vi "final with visa and without stepper motor.vi"() -> ()   [LabVIEW 2022 SP3]
uses:
  <vilib>/DAQmx/create/channels.llb/DAQmx Create Channel (AI-Voltage-Basic).vi
  <vilib>/DAQmx/read.llb/DAQmx Read (Analog 1D DBL NChan 1Samp).vi
panel:
  in  "VISA resource name 2":refnum<visa-resource-name>
  in  "VISA resource name":refnum<visa-resource-name>
  in  "physical channels":tag
  in  "stop":bool
  out "humidity":dbl
  in  "Voltage":dbl
  out "?":bool
  out "Counter":dbl
  out "number":dbl
  out "weight":dbl
  out "voltage (weight)":dbl
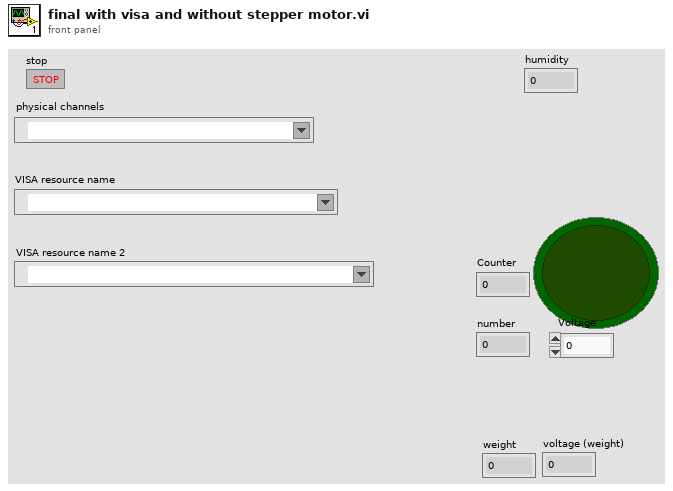
[diagram p1: front panel]
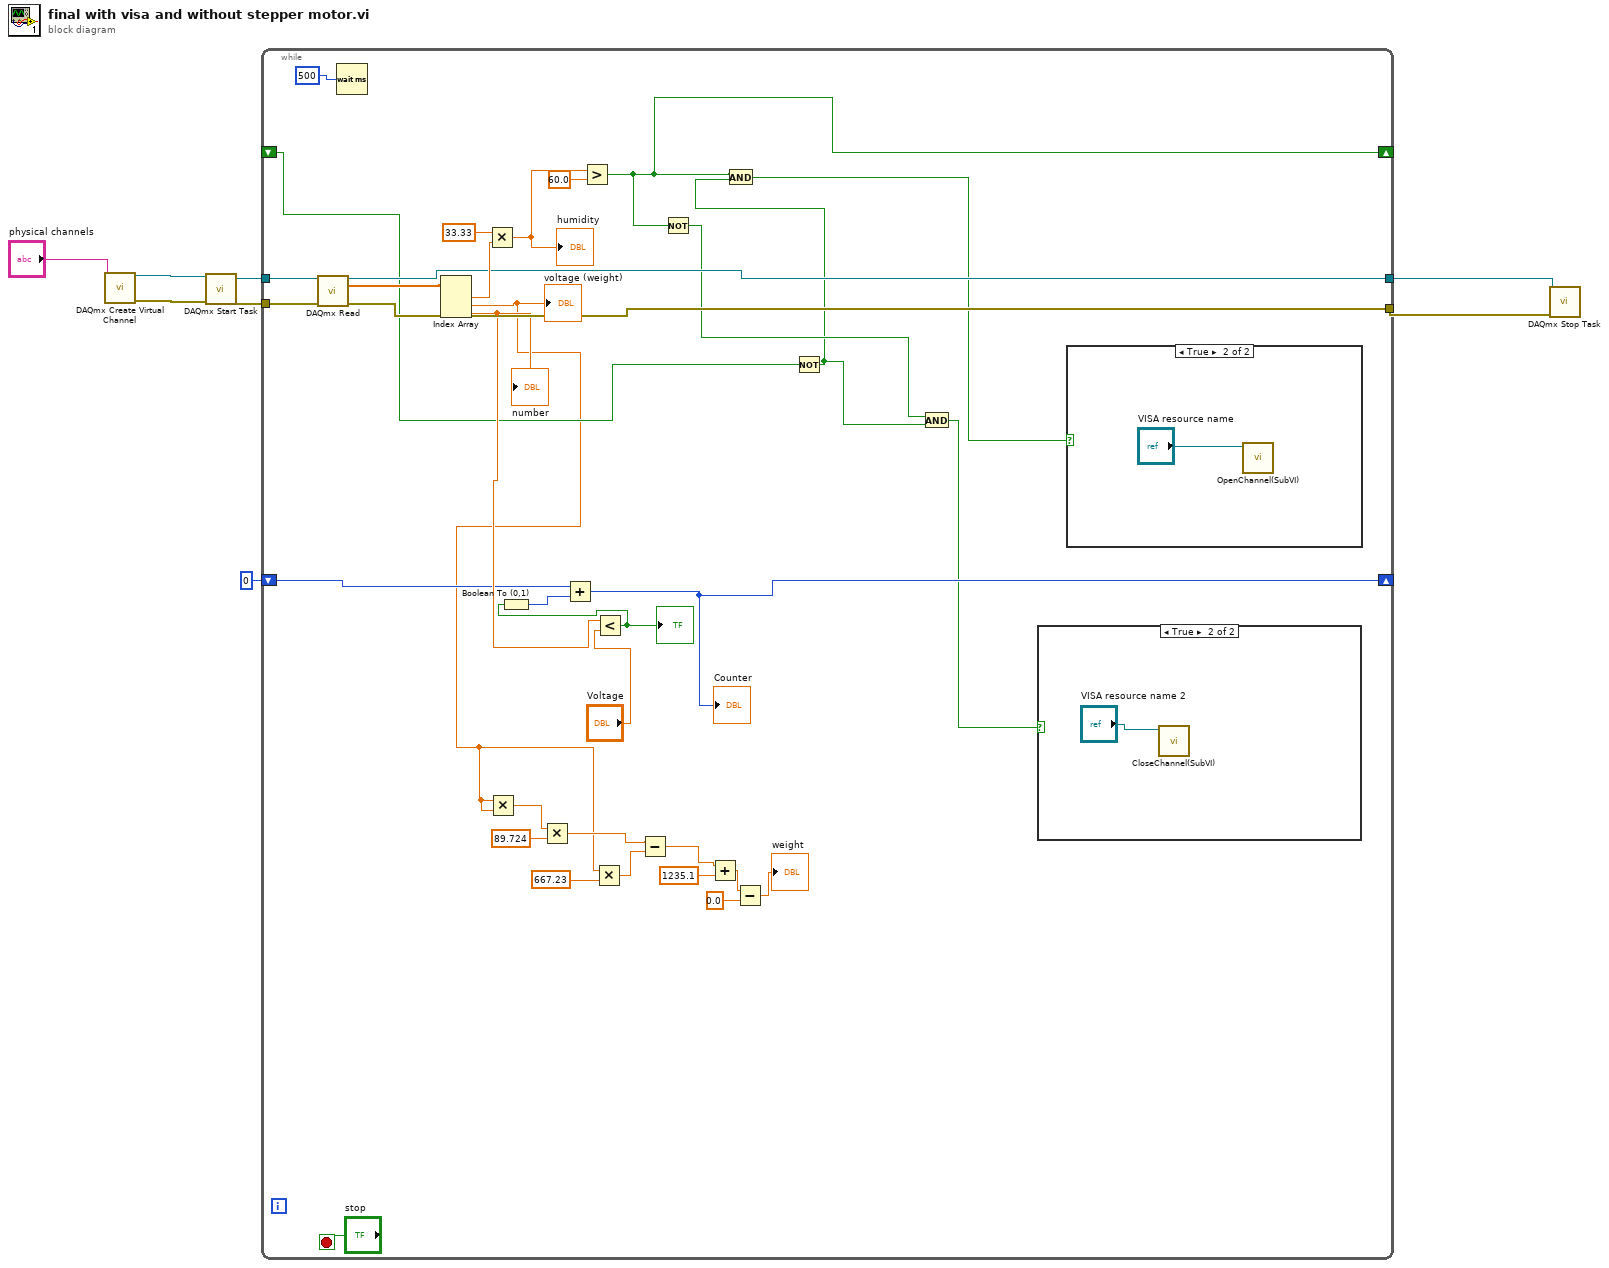
[diagram p0: block diagram]
diagram:
  n1 = call-poly <vilib>:"DAQmx Create Virtual Channel.vi"("physical channels"="physical channels") -> ("task out"=w8:refnum<k21>, "error out"=w7:errorcluster)  [unwired: 13 in]
  n2 = call <vilib>:"DAQmx Start Task.vi"("task/channels in"=w8, "error in"=w7) -> ("task out"=w6:refnum<k21>, "error out"=w5:errorcluster)  [unwired: 12 in]
  n3 = while {
    tunnel: w6 -> [w42]
    tunnel: w5 -> [w41]
    tunnel: [w33] -> w4
    tunnel: [w34] -> w2
    shift-right: [w28] -> _
    shift-left: i16 0 -> [w27]
    shift-right: [w17] -> _
    shift-left: _ -> [w15]
    stop <- "stop" stop-if-true
    n4 = call-poly <vilib>:"DAQmx Read.vi"("task/channels in"=w42, "error in"=w41) -> ("task out"=w33:refnum<k21>, "data"=w38:dbl[], "error out"=w34:errorcluster)  [unwired: 11 in]
    n5 = Wait (ms)(milliseconds to wait=u32 500) -> ()  [unwired: 1 out]
    n6 = Index Array(array=w38) -> (element #1=w37:dbl, element #2=w10:dbl, element #3=w29:dbl)  [unwired: 3 in]
    "number" <- w29
    "voltage (weight)" <- w10
    n7 = Multiply(x=33.33, y=w37) -> (x*y=w11:dbl)
    "humidity" <- w11
    n8 = Multiply(x=w10, y=w10) -> (x*y=w9:dbl)
    n9 = Multiply(x=w9, y=89.724) -> (x*y=w24:dbl)
    n10 = Greater?(x=w11, y=60.0) -> (0:w17:bool)
    n11 = Multiply(x=w10, y=667.23) -> (x*y=w23:dbl)
    n12 = Less?(x=w29, y="Voltage") -> (x < y?=w30:bool)
    "?" <- w30
    n13 = Boolean To (0,1)(Boolean=w30) -> (0, 1=w31:i16)
    n14 = Add(x=w27, y=w31) -> (x+y=w28:i16)
    "Counter" <- w28
    n15 = Subtract(x=w24, y=w23) -> (x-y=w21:dbl)
    n16 = Not(x=w17) -> (.not. x?=w16:bool)
    n17 = Add(x=w21, y=1235.1) -> (x+y=w19:dbl)
    n18 = Subtract(x=w19, y=0.0) -> (x-y=→"weight":dbl)
    n19 = Not(x=w15) -> (.not. x?=w12:bool)
    n20 = And(x=w17, y=w12) -> (x .and. y?=w14:bool)
    n21 = And(x=w16, y=w12) -> (x .and. y?=w13:bool)
    n22 = case shown="True" w13 {
      frame False {
      }
      frame True {
        n23 = call "CloseChannel(SubVI).vi"("VISA Refnum in"="VISA resource name 2") -> ()  [unwired: 11 in]
      }
    }
    n24 = case shown="True" w14 {
      frame False {
      }
      frame True {
        n25 = call "OpenChannel(SubVI).vi"("VISA Refnum in"="VISA resource name") -> ()  [unwired: 11 in]
      }
    }
  }
  n26 = call <vilib>:"DAQmx Stop Task.vi"("task/channels in"=w4, "error in"=w2) -> ()  [unwired: 12 in, 2 out]
